vi "test Fails If Seconds Are Not Equal.vi"(8 "error in (no error)":errorcluster, 11 "TestCase in":refnum<class "Timestamp Comparison Test Case.lvclass">) -> (0 "error out":errorcluster, 3 "TestCase out":refnum<class "Timestamp Comparison Test Case.lvclass">)   [LabVIEW 2015, in "Timestamp Comparison Test Case.lvclass"]
uses:
  Timestamp Comparison Test Case.lvclass
  <vilib>/addons/_JKI Toolkits/VI Tester/TestCase.llb/TestCase.lvclass
  VITAC.lvlib
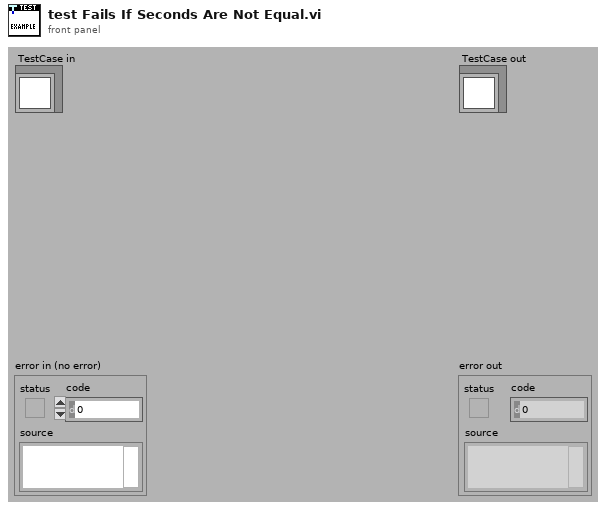
[diagram p1: front panel]
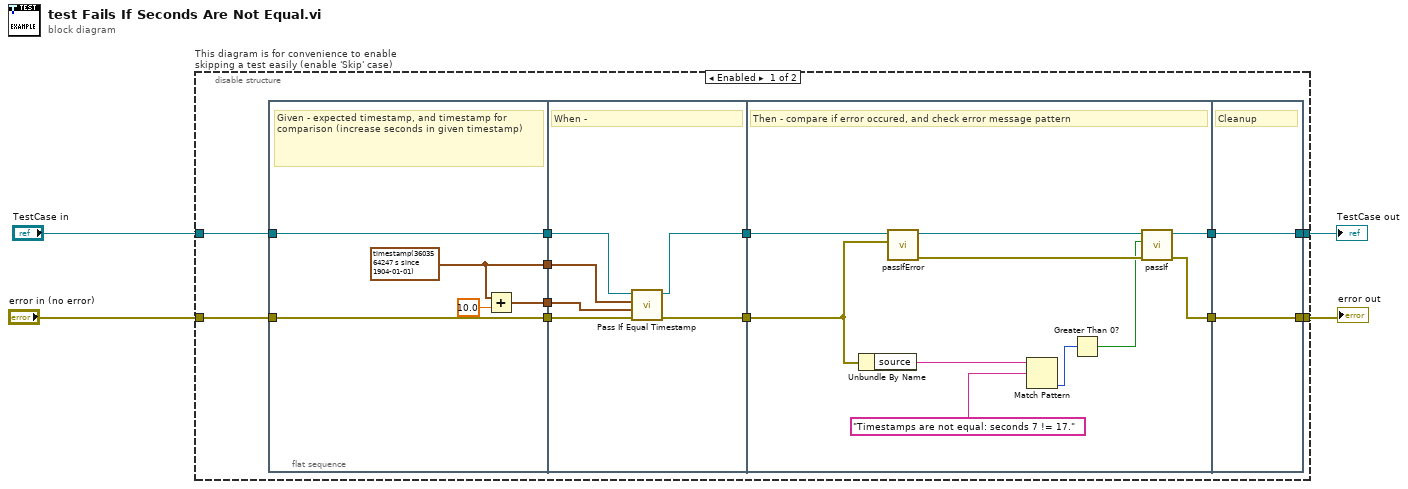
[diagram p0: block diagram]
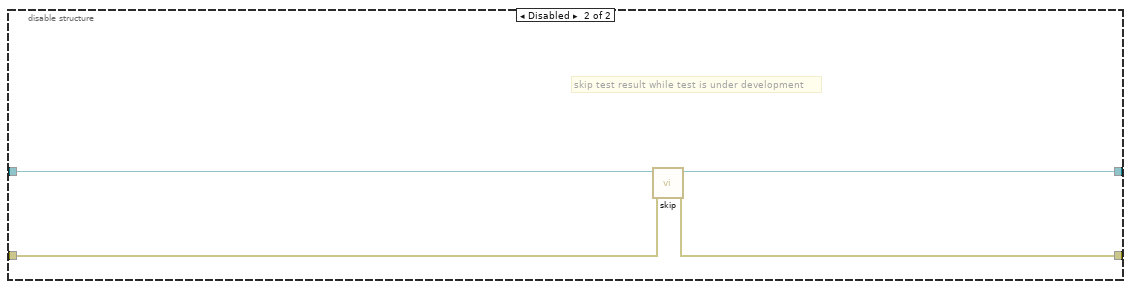
[diagram p2: hidden frame]
diagram:
  n1 = disable-structure "This diagram is for convenience to enable skipping a test easily (enable 'Skip' case)" shown="Enabled" {
    disable-tunnel: "TestCase in" -> [w8 w43]
    disable-tunnel: [w10 w41] -> w1
    disable-tunnel: [w9 w42] -> w3
    disable-tunnel: "error in (no error)" -> [w7 w40]
    frame Enabled {
      n2 = flat-sequence {
        tunnel: w7 -> [w20]
        tunnel: w8 -> [w21]
        tunnel: [w21] -> w16
        tunnel: [w20] -> w15
        tunnel: [w19] -> w6
        tunnel: [w17] -> w5
        tunnel: [w24] -> w14
        tunnel: [w26] -> w13
        tunnel: w16 -> [w25]
        tunnel: w15 -> [w27]
        tunnel: w6 -> [w23]
        tunnel: w5 -> [w22]
        tunnel: [w28] -> w12
        tunnel: w14 -> [w31]
        tunnel: w13 -> [w30]
        tunnel: [w29] -> w11
        tunnel: [w38] -> w9
        tunnel: [w39] -> w10
        tunnel: w12 -> [w39]
        tunnel: w11 -> [w38]
        frame #0 {
          w19 = timestamp(3603564247.1 s since 1904-01-01) ("current time")
          # "Given - expected timestamp, and timestamp for comparison (increase seconds in given timestamp)"
          n3 = Add(x=w19, y=10.0) -> (x+y=w17:timestamp)
        }
        frame #1 {
          # "When -"
          n4 = call "Pass If Equal Timestamp.vi"("error in (no error)"=w27, "actual timestamp"=w22, "expected timestamp"=w23, "TestCase in"=w25) -> ("error out"=w26:errorcluster, "TestCase out"=w24:refnum<class "Timestamp Comparison Test Case.lvclass">)  [unwired: 6 in]
        }
        frame #2 {
          # "Then - compare if error occured, and check error message pattern"
          n5 = Unbundle By Name(w30) -> ("source"=w35:string)
          n6 = call-dynamic "passIfError.vi"("error"=w30, "TestCase in"=w31) -> ("error out"=w36:errorcluster, "TestCase out"=w37:refnum<class "Timestamp Comparison Test Case.lvclass">)  [unwired: 8 in]
          n7 = Match Pattern(string=w35, regular expression="Timestamps are not equal: seconds 7 != 17.") -> (offset past match=w33:i32)  [unwired: 1 in, 3 out]
          n8 = Greater Than 0?(x=w33) -> (x > 0?=w32:bool)
          n9 = call-dynamic "passIf.vi"("error in (no error)"=w36, "pass"=w32, "TestCase in"=w37) -> ("error out"=w29:errorcluster, "TestCase out"=w28:refnum<class "Timestamp Comparison Test Case.lvclass">)  [unwired: 7 in]
        }
        frame #3 {
          # "Cleanup"
        }
      }
    }
    frame Disabled {
      # "skip test result while test is under development"
      n10 = call <vilib>:"skip.vi"("error in (no error)"=w40, "TestCase in"=w43) -> ("error out"=w42:errorcluster, "TestCase out"=w41:refnum<class "Timestamp Comparison Test Case.lvclass">)  [unwired: 8 in]
    }
  }
  "error out" <- w3
  "TestCase out" <- w1
